vi "CreateImages.vi"(8 "error in (no error)":errorcluster, 10 "Array 3":T1[](array[typedef]) items=["Grayscale (U8)", "Grayscale (I16)", "Grayscale (SGL)", "Complex (CSG)", "RGB (U32)", "HSL (U32)", "RGB (U64)", "Grayscale (U16)"], 11 "Array in":string[](array[string])) -> (0 "error in (no error) 2":errorcluster, 3 "Array out":T2[](array[typedef]))   [LabVIEW 2022 SP3]
uses:
  Classes/DLP2/DLP2.lvclass/DLP2.ctl
  <vilib>/vision/Image Controls.llb/IMAQ Image.ctl
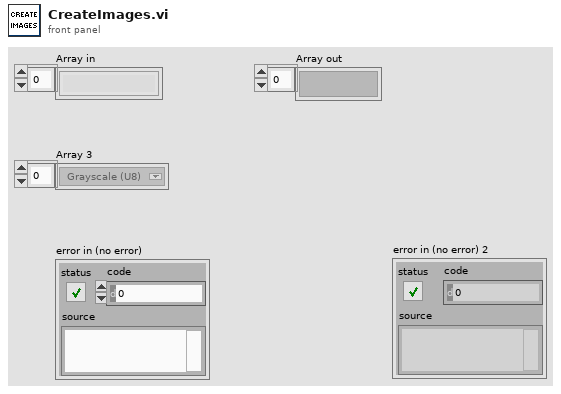
[diagram p1: front panel]
types:
  T1 = typedef "Image Type" = u32
  T2 = typedef "IMAQ Image.ctl" = refnum<image>
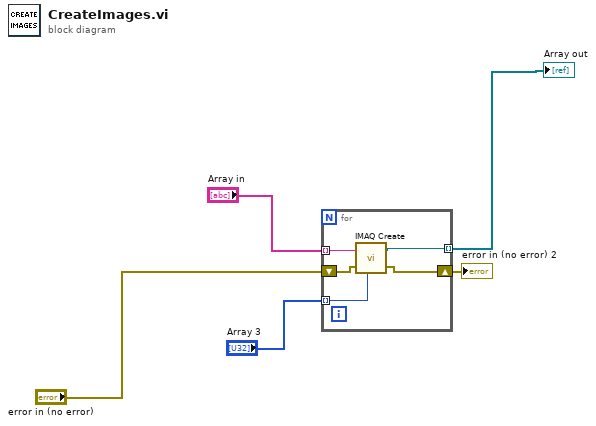
[diagram p0: block diagram]
diagram:
  n1 = for {
    tunnel: "Array 3" -> [w10] mode=indexing
    tunnel: "Array in" -> [w9] mode=indexing
    tunnel: [w8] -> w5 mode=indexing
    shift-right: [w6] -> w1
    shift-left: "error in (no error)" -> [w7]
    n2 = call "IMAQ Create"("Image Name"=w9, "Image Type"=w10, "error in (no error)"=w7) -> ("New Image"=w8:T2, "error out"=w6:errorcluster)  [unwired: 2 in]
  }
  "Array out" <- w5
  "error in (no error) 2" <- w1
